vi "Raw Text to 1D String.vi"(8 "Error In":errorcluster, 9 "Use Example Input":bool, 10 "Example Input":string, 11 "Relative Path to Input File":string) -> (0 "Error Out":errorcluster, 3 "1D String Array":string[](array[string]))   [LabVIEW 2019]
doc: "Given a relative path, retrieve a 1D string array from an input text file. This assumes Line Feed delimiters."
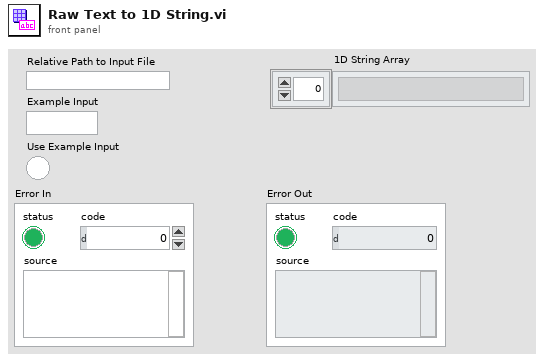
[diagram p1: front panel]
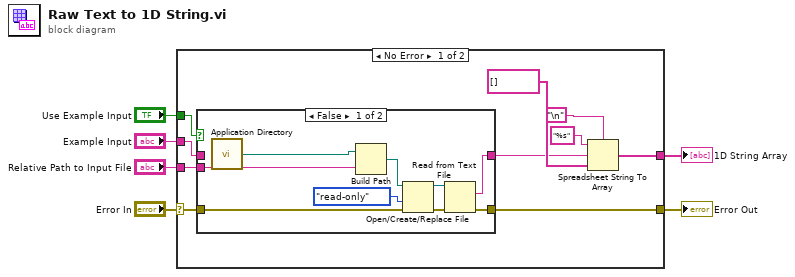
[diagram p0: block diagram]
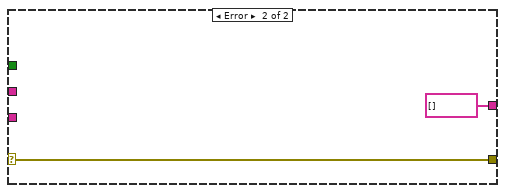
[diagram p3: hidden frame]
diagram:
  n1 = case shown="No Error" "Error In" {
    selector: "Error In" -> [w9 w29]
    tunnel: "Relative Path to Input File" -> [w16 _]
    tunnel: [w12 string[] []] -> w5
    tunnel: [w11 w29] -> w4
    tunnel: "Use Example Input" -> [w8 _]
    tunnel: "Example Input" -> [w7 _]
    frame No Error {
      n2 = case shown="False" w8 {
        tunnel: w16 -> [w24 _]
        tunnel: [w19 w27] -> w14
        tunnel: [w18 w26] -> w11
        tunnel: w9 -> [w17 w26]
        tunnel: w7 -> [_ w27]
        frame False {
          n3 = call <vilib>:"Application Directory.vi"() -> ("Application Directory"=w25:path)
          n4 = Build Path(base path=w25, name or relative path=w24) -> (appended path=w23:path)
          n5 = Open/Create/Replace File(file path (use dialog)=w23, error in=w17, access (0:read/write)=enum16{"read/write", "read-only", "write-only"}."read-only") -> (refnum out=w21:refnum<file>, error out=w20:errorcluster)  [unwired: 3 in, 1 out]
          n6 = Read from Text File(file (use dialog)=w21, error in=w20) -> (text=w19:string, error out=w18:errorcluster)  [unwired: 2 in, 2 out]
        }
        frame True {
        }
      }
      n7 = Spreadsheet String To Array(delimiter (Tab)="\n", format string="%s", spreadsheet string=w14, array type (2D Dbl)=string[] []) -> (array=w12:string[])
    }
    frame Error {
    }
  }
  "Error Out" <- w4
  "1D String Array" <- w5
